vi "Test Parsing Simple Example Test 1.vi"() -> ()   [LabVIEW 2014]
uses:
  <vilib>/Utility/traverseref.llb/TRef TravTarget.ctl
  <vilib>/Utility/traverseref.llb/VI Scripting - Traverse.lvlib
panel:
  out "SubVI C calls":string[](array[string])
  out "error wires info":T1
  in  "vi path":path=path "C:/Users/lubo/Documents/LabView/LabVIEW-Universal-Transcriptor/Test/Examples For Parsing/Example Test 1.vi"
  # "This is here just for debug, for now I'm going to scan error wires and transcript VI on it to some C call functions."
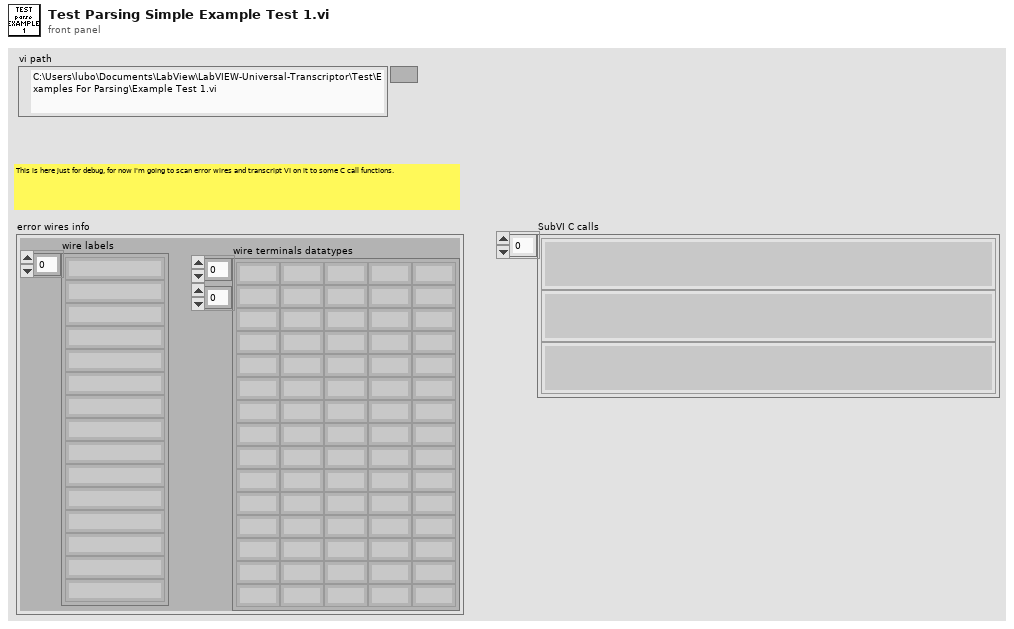
[diagram p1: front panel]
types:
  T1 = cluster{"wire labels":string[], "wire terminals datatypes":string[][]}
  T2 = typedef "TRef TravTarget.ctl" = enum16{"FP", "BD", "Other"}
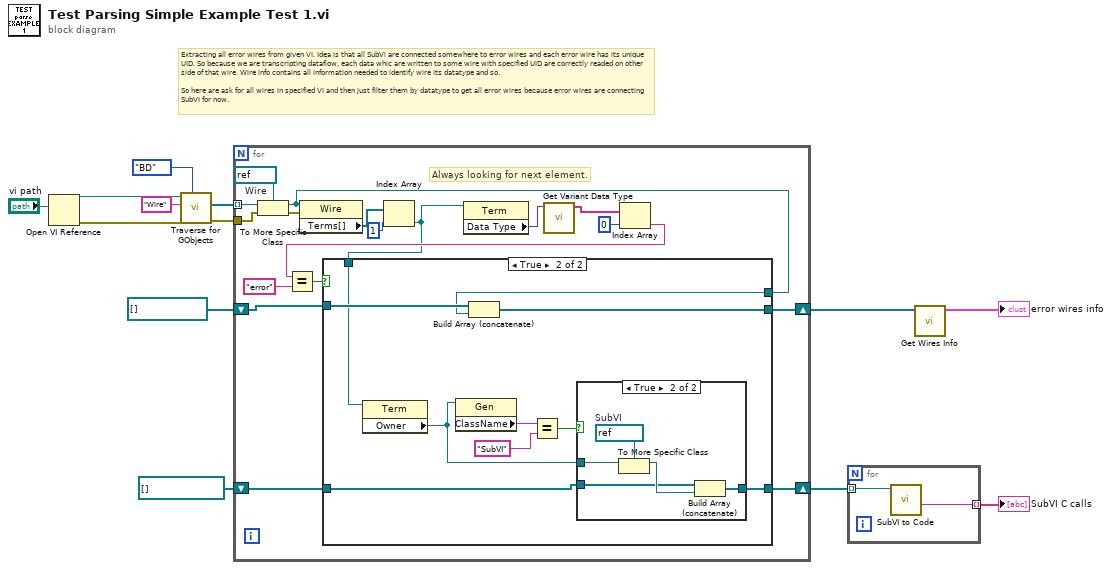
[diagram p0: block diagram]
diagram:
  # "Extracting all error wires from given VI. Idea is that all SubVi are connected somewhere to error wires and each error wire has its unique UID. So because we are transcripting dataflow, each data whic are written to some wire with specified UID are correctly readed on other side of that wire. Wire info contains all information needed to identify wire its datatype and so.\n\nSo here are ask for all wires in specified VI and then just filter them by datatype to get all error wires because error wires are connecting SubVI for now."
  n1 = Open VI Reference(vi path="vi path") -> (vi reference=w12:refnum<vi>, error out=w9:errorcluster)  [unwired: 5 in]
  n2 = call <vilib>:"Traverse for GObjects.vi"("Traverse Target"=TRef_TravTarget."BD", "error in (no error)"=w9, "Class Name"="Wire", "VI Refnum"=w12) -> ("error out"=w7:errorcluster, "References"=w8:refnum<vi>[])  [unwired: 4 in, 2 out]
  n3 = for {
    tunnel: w8 -> [w21] mode=indexing
    tunnel: w7 -> [w31]
    shift-right: [w19] -> w5
    shift-left: refnum<vi>[] [] -> [w18]
    shift-right: [w16] -> w2
    shift-left: refnum<vi>[] [] -> [w15]
    w30 = refnum<vi> refnum  # Wire
    # "Always looking for next element."
    n4 = To More Specific Class(target class=w30, reference=w21, error in=w31) -> (specific class reference=w20:refnum<vi>, error out=w29:errorcluster)
    n5 = property class="Wire"(reference=w20, error in=w29) -> ("Terms[]"=w28:refnum<vi>[])  [unwired: 2 out]
    n6 = Index Array(array=w28, index=1) -> (element=w14:refnum<vi>)
    n7 = property class="Term"(reference=w14) -> ("Data Type"=w27:variant)  [unwired: 1 in, 2 out]
    n8 = call "Get Variant Data Type.vi"("variant"=w27) -> ("Data Type"=w26:string[])  [unwired: 10 in]
    n9 = Index Array(array=w26, index=0) -> (element=w24:string)
    n10 = Equal?(x=w24, y="error") -> (x = y?=w17:bool)
    n11 = case shown="True" w17 {
      tunnel: w20 -> [_ w34]
      tunnel: [w33 w43] -> w19
      tunnel: w18 -> [w33 w42]
      tunnel: [w32 w37] -> w16
      tunnel: w15 -> [w32 w36]
      tunnel: w14 -> [_ w35]
      frame False {
      }
      frame True {
        n12 = property class="Term"(reference=w35) -> ("Owner"=w41:refnum<vi>)  [unwired: 1 in, 2 out]
        n13 = property class="Gen"(reference=w41) -> ("ClassName"=w38:string)  [unwired: 1 in, 2 out]
        n14 = Build Array (concatenate)(w42, w34) -> (w43:refnum<vi>[])
        n15 = Equal?(x=w38, y="SubVI") -> (x = y?=w40:bool)
        n16 = case shown="True" w40 {
          tunnel: w41 -> [_ w48]
          tunnel: [w44 w45] -> w37
          tunnel: w36 -> [w44 w46]
          frame False {
          }
          frame True {
            w49 = refnum<vi> refnum  # SubVI
            n17 = To More Specific Class(target class=w49, reference=w48) -> (specific class reference=w47:refnum<vi>)  [unwired: 1 in, 1 out]
            n18 = Build Array (concatenate)(w46, w47) -> (w45:refnum<vi>[])
          }
        }
      }
    }
  }
  n19 = for {
    tunnel: w2 -> [w51] mode=indexing
    tunnel: [w50] -> w1 mode=indexing
    n20 = call "SubVI to Code.vi"("reference"=w51) -> ("SubVI C call"=w50:string)  [unwired: 8 in, 2 out]
  }
  "SubVI C calls" <- w1
  n21 = call "Get Wires Info.vi"("connected\nwires refs."=w5) -> ("output cluster 2"=→"error wires info":T1)  [unwired: 10 in]
